vi "U3 I2C EEPROM.vi"() -> ()   [LabVIEW 2021]
panel:
  out "U8 Array Read":u8[](array[numeric])
  in  "U8 Array Write":u8[](array[numeric])=[170, 240, 170, 240]
  out "Error Message":string
  out "error out":errorcluster
  # "I2C example uses the first found USB device.  Writes and reads bytes from the user\narea (0-63) of the 24C01C EEPROM on the LJTick-DAC, which is plugged into FIO4/FIO5.\n\nTested with UD V2.73 and U3 firmware V1.40."
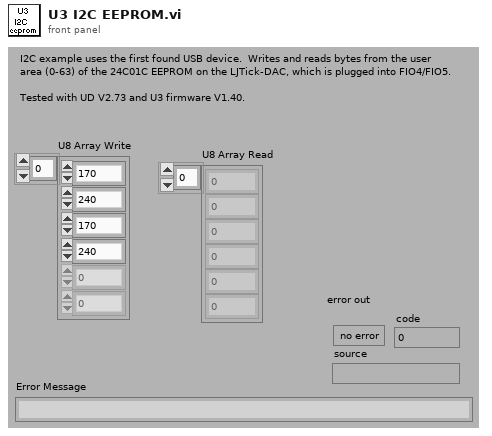
[diagram p1: front panel]
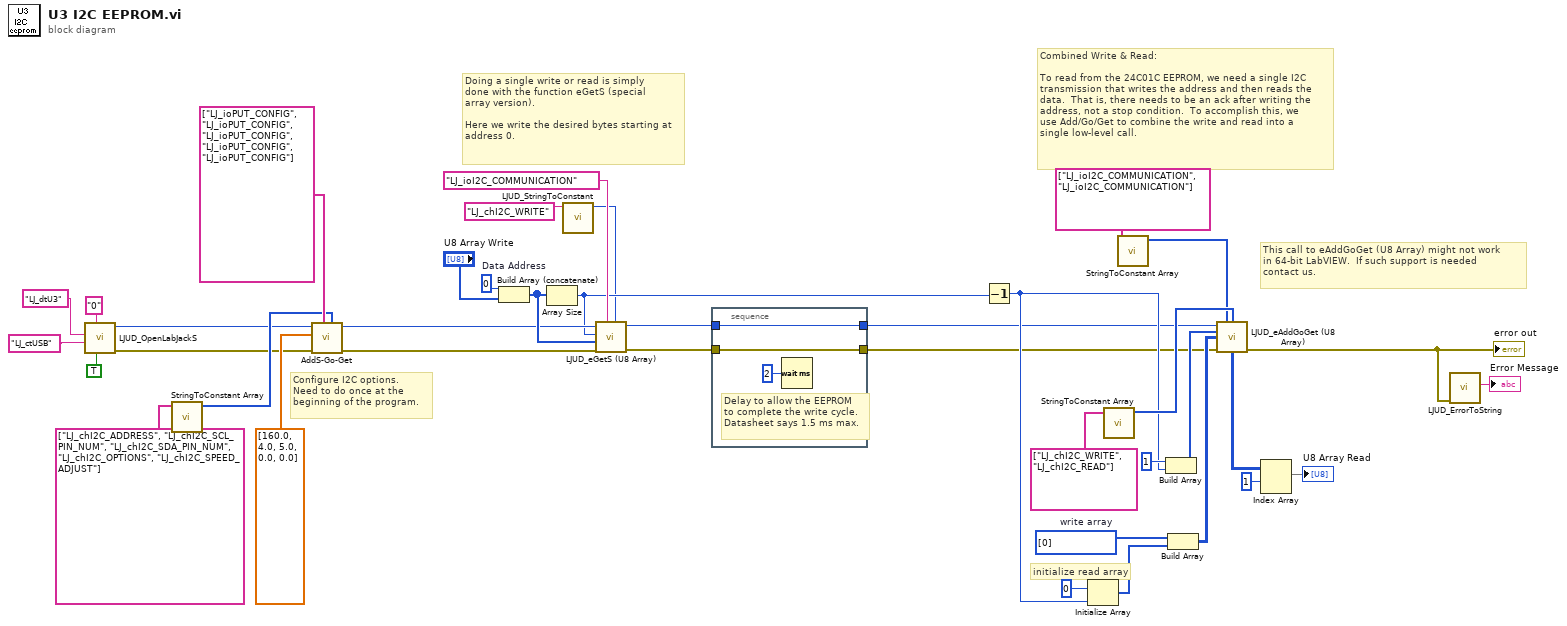
[diagram p0: block diagram]
diagram:
  w12 = u8[] [0]  # write array
  w23 = u8 0  # Data Address
  # "This call to eAddGoGet (U8 Array) might not work\nin 64-bit LabVIEW.  If such support is needed\ncontact us."
  # "Combined Write & Read:\n\nTo read from the 24C01C EEPROM, we need a single I2C\ntransmission that writes the address and then reads the\ndata.  That is, there needs to be an ack after writing the\naddress, not a stop condition.  To accomplish this, we\nuse Add/Go/Get to combine the write and read into a\nsingle low-level call."
  # "initialize read array"
  # "Doing a single write or read is simply\ndone with the function eGetS (special\narray version).  \n\nHere we write the desired bytes starting at\naddress 0."
  # "Configure I2C options.\nNeed to do once at the\nbeginning of the program."
  n1 = call "LJUD_OpenLabJackS.vi"("FirstFound"=TRUE, "Address"="0", "ConnectionType"="LJ_ctUSB", "DeviceType"="LJ_dtU3") -> ("error out"=w29:errorcluster, "Handle"=w28:i32)  [unwired: 5 in, 1 out]
  n2 = call "StringToConstant Array.vi"("String Constant Array In"=string[] ["LJ_chI2C_ADDRESS", "LJ_chI2C_SCL_PIN_NUM", "LJ_chI2C_SDA_PIN_NUM", "LJ_chI2C_OPTIONS", "LJ_chI2C_SPEED_ADJUST"] ("IOTypes")) -> ("I32 Constant Array Out"=w30:i32[])  [unwired: 10 in]
  n3 = call "AddS-Go-Get.vi"("Channels"=w30, "IOTypes"=string[] ["LJ_ioPUT_CONFIG", "LJ_ioPUT_CONFIG", "LJ_ioPUT_CONFIG", "LJ_ioPUT_CONFIG", "LJ_ioPUT_CONFIG"], "error in"=w29, "Values Write"=dbl[] [160.0, 4.0, 5.0, 0.0, 0.0], "Handle In"=w28) -> ("error out"=w26:errorcluster, "Handle Out"=w25:i32)  [unwired: 4 in, 1 out]
  n4 = Build Array (concatenate)(w23, "U8 Array Write") -> (w27:u8[])
  n5 = Array Size(array=w27) -> (size(s)=w20:i32)
  n6 = call "LJUD_StringToConstant.vi"("String"="LJ_chI2C_WRITE" ("IOType")) -> ("Constant Number"=w6:i32)  [unwired: 9 in, 1 out]
  n7 = call "LJUD_eGetS (U8 Array).vi"("Channel"=w6, "IOType"="LJ_ioI2C_COMMUNICATION", "error in"=w26, "U8 Array Write"=w27, "Value"=w20, "Handle In"=w25) -> ("error out"=w4:errorcluster, "Handle Out"=w2:i32)  [unwired: 2 in, 2 out]
  n8 = stacked-sequence {
    tunnel: w4 -> [w42]
    tunnel: [w42] -> w3
    tunnel: w2 -> [w41]
    tunnel: [w41] -> w1
    frame #0 {
      # "Delay to allow the EEPROM\nto complete the write cycle.\nDatasheet says 1.5 ms max."
      n9 = Wait (ms)(milliseconds to wait=u32 2) -> ()  [unwired: 1 out]
    }
  }
  n10 = Decrement(x=w20) -> (x-1=w14:i32)
  n11 = Initialize Array(u8 0 ("Element Data"), w14) -> (w11:u8[])
  n12 = call "StringToConstant Array.vi"("String Constant Array In"=string[] ["LJ_chI2C_WRITE", "LJ_chI2C_READ"] ("IOTypes")) -> ("I32 Constant Array Out"=w17:i32[])  [unwired: 10 in]
  n13 = call "StringToConstant Array.vi"("String Constant Array In"=string[] ["LJ_ioI2C_COMMUNICATION", "LJ_ioI2C_COMMUNICATION"] ("IOTypes")) -> ("I32 Constant Array Out"=w16:i32[])  [unwired: 10 in]
  n14 = Build Array(1 ("Input Element"), w14) -> (w18:i32[])
  n15 = Build Array(w12, w11) -> (w15:u8[][])
  n16 = call "LJUD_eAddGoGet (U8 Array).vi"("Handle In"=w1, "aIOTypes"=w16, "aChannels"=w17, "Values Write"=w18, "ax1s Write (U8 Arrays)"=w15, "error in"=w3) -> ("ax1s Read (U8 Arrays)"=w10:u8[][], "error out"=w22:errorcluster)  [unwired: 3 in, 5 out]
  "error out" <- w22
  n17 = Index Array(array=w10, index (row)=1 ("Index (row)")) -> (element=→"U8 Array Read":u8[])  [unwired: 1 in]
  n18 = call "LJUD_ErrorToString.vi"("error in"=w22) -> ("String"=→"Error Message":string)  [unwired: 10 in]
